vi "Rcv Cmd.vi"(8 "error in":errorcluster, 11 "eCRDS in":refnum<class "eCRDS.lvclass">) -> (0 "error out":errorcluster, 3 "eCRDS out":refnum<class "eCRDS.lvclass">)   [LabVIEW 2014, in "eCRDS Library.lvlib" / "eCRDS.lvclass"]
uses:
  eCRDS.lvclass
  eCRDS.lvclass/eCRDS.ctl
  reusable/Instrument/Instrument.lvclass/Instrument.ctl
  reusable/CRDS/Data/Main/CRDS Data.lvclass
  reusable/CRDS/Cell/CRDS Cell.lvclass/CRDS Cell.ctl
  reusable/CRDS/Cell/Read Data.vi
  reusable/CRDS/Cell/Write Data.vi
  Accessors/Read HK DVR.vi
  reusable/Instrument/Read Data.vi
  reusable/Instrument/Write Data.vi
  reusable/CRDS/Main/Write Cells.vi
  reusable/CRDS/Data/Main/Write CellData.vi
  reusable/CRDS/Data/Cell/Write hkParam.vi
  reusable/CRDS/Data/Cell/Read hkParam.vi
  reusable/CRDS/Data/Main/Read CellData.vi
  reusable/CRDS/Main/Read Cells.vi
  reusable/CRDS/Data/Cell/CRDS Cell Data.lvclass
  reusable/CRDS/Cell/CRDS Cell.lvclass
  reusable/Data/Data.lvlibp/Data.lvclass
  reusable/CRDS/Main/CRDS.lvclass
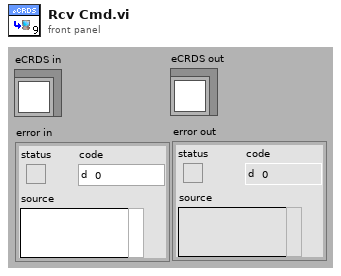
[diagram p1: front panel]
types:
  T1 = cluster{"T (degC)":dbl, "P (mb)":dbl, "Q (lpm)":dbl}[]
  T2 = typedef "hkParam Ctl.ctl" = cluster{"rhDilFac":sgl, "Q":sgl, "Tmean":sgl, "extDilFac":sgl, "rhCell":sgl, "P":sgl, "T":sgl}
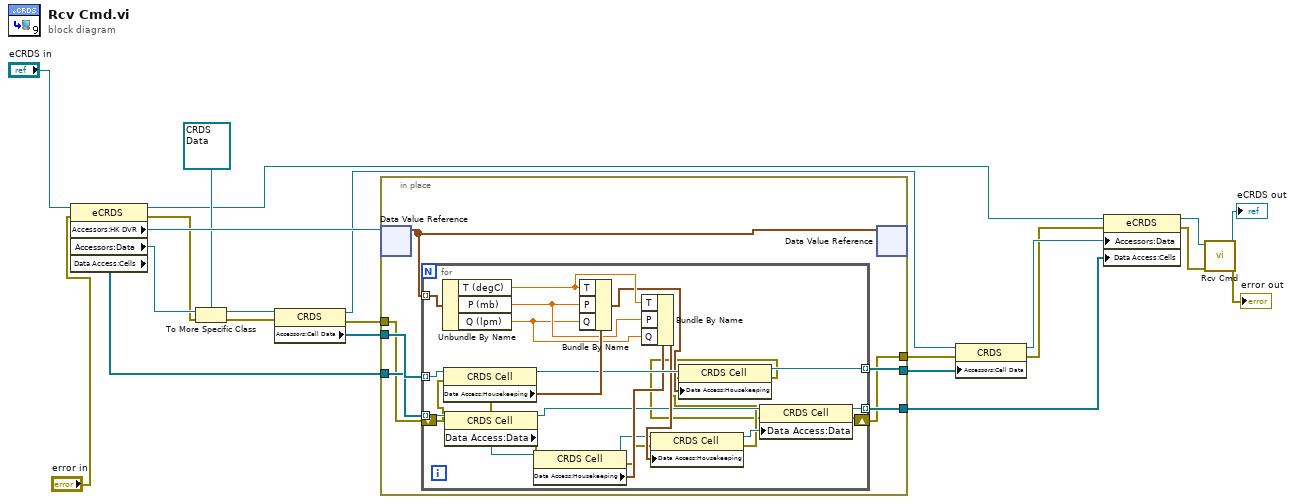
[diagram p0: block diagram]
diagram:
  n1 = property class="eCRDS"(reference="eCRDS in", error in="error in") -> (reference out=w13:refnum<class "eCRDS.lvclass">, error out=w9:errorcluster, "Accessors:HK DVR"=w21:refnum<data-value>, "Accessors:Data"=w20:refnum<class "Data.lvclass">, "Data Access:Cells"=w16:refnum<class "CRDS Cell.lvclass">[])
  n2 = To More Specific Class(target class=refnum<class "CRDS Data.lvclass"> refnum ("CRDS Lib.lvlib:CRDS"), reference=w20, error in=w9) -> (specific class reference=w18:refnum<class "CRDS Data.lvclass">, error out=w8:errorcluster)
  n3 = property class="CRDS"(reference=w18, error in=w8) -> (reference out=w15:refnum<class "CRDS Data.lvclass">, error out=w7:errorcluster, "Accessors:Cell Data"=w17:refnum<class "CRDS Cell Data.lvclass">[])
  n4 = in-place {
    in-place-border: w17 -> [w29]
    in-place-border: w16 -> [w28]
    in-place-border: [w26] -> w14
    in-place-border: [w25] -> w11
    in-place-border: w7 -> [w24]
    in-place-border: [w23] -> w6
    n5 = in-place-dvr #1(w21) -> (w27:T1)  [unwired: 1 out]
    n6 = for {
      tunnel: w29 -> [w52] mode=indexing
      tunnel: w28 -> [w50] mode=indexing
      tunnel: w27 -> [w53] mode=indexing
      tunnel: [w41] -> w26 mode=indexing
      tunnel: [w38] -> w25 mode=indexing
      shift-right: [w31] -> w23
      shift-left: w24 -> [w37]
      n7 = Unbundle By Name(w53) -> ("T (degC)"=w46:dbl, "P (mb)"=w45:dbl, "Q (lpm)"=w44:dbl)
      n8 = property class="CRDS Cell"(reference=w52, error in=w37) -> (reference out=w49:refnum<class "CRDS Cell Data.lvclass">, error out=w36:errorcluster, "Data Access:Housekeeping"=w51:T2)
      n9 = property class="CRDS Cell"(reference=w50, error in=w36) -> (reference out=w39:refnum<class "CRDS Cell.lvclass">, error out=w35:errorcluster, "Data Access:Data"=w48:refnum<class "CRDS Cell Data.lvclass">)
      n10 = property class="CRDS Cell"(reference=w48, error in=w35) -> (reference out=w30:refnum<class "CRDS Cell Data.lvclass">, error out=w34:errorcluster, "Data Access:Housekeeping"=w47:T2)
      n11 = Bundle By Name(cluster=w51, "T"=w46, "P"=w45, "Q"=w44) -> (w42:T2)
      n12 = Bundle By Name(cluster=w47, "T"=w46, "P"=w45, "Q"=w44) -> (w43:T2)
      n13 = property class="CRDS Cell"(reference=w30, error in=w34, "Data Access:Housekeeping"=w43) -> (reference out=w40:refnum<class "CRDS Cell Data.lvclass">, error out=w33:errorcluster)
      n14 = property class="CRDS Cell"(reference=w49, error in=w33, "Data Access:Housekeeping"=w42) -> (reference out=w41:refnum<class "CRDS Cell Data.lvclass">, error out=w32:errorcluster)
      n15 = property class="CRDS Cell"(reference=w39, error in=w32, "Data Access:Data"=w40) -> (reference out=w38:refnum<class "CRDS Cell.lvclass">, error out=w31:errorcluster)
    }
    n16 = in-place-dvr #1(w27) -> ()  [unwired: 2 out]
  }
  n17 = property class="CRDS"(reference=w15, error in=w6, "Accessors:Cell Data"=w14) -> (reference out=w12:refnum<class "CRDS Data.lvclass">, error out=w5:errorcluster)
  n18 = property class="eCRDS"(reference=w13, error in=w5, "Accessors:Data"=w12, "Data Access:Cells"=w11) -> (reference out=w4:refnum<class "eCRDS.lvclass">, error out=w2:errorcluster)
  n19 = call-parent "Rcv Cmd.vi"("error in"=w2, "Instrument in"=w4) -> ("error out"=→"error out":errorcluster, "Instrument out"=→"eCRDS out":refnum<class "eCRDS.lvclass">)  [unwired: 8 in]
